vi "MoveCarriageToPosition.vi"(6 "Lift Speed":dbl, 7 "Target Height":dbl) -> ()   [LabVIEW 2017]
uses:
  Robot Global Data.vi
  <vilib>/Rock Robotics/Network Tables/NT Write Number.vi
  <vilib>/addons/control/pid/pid.llb/PID (DBL).vi
  <vilib>/addons/control/pid/NI_PID_pid.lvlib
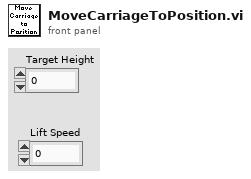
[diagram p1: front panel]
types:
  T1 = cluster{"proportional gain (Kc)":dbl, "integral time (Ti, min)":dbl, "derivative time (Td, min)":dbl}
  T2 = typedef "WPI_MotorControlDeviceRef.ctl" = cluster{"DeviceStatus":errorcluster, "Type":T3, "PWM":cluster{"PWM Channel":T4, "DeadBand":T5}, "CAN":cluster{"Device Number":u8, "SetOutput VI Ref":variant, "GetOutput VI Ref":variant, "Enable VI Ref":variant, "Disable VI Ref":variant, "Data":variant}, "Invert":bool, "DIO PWM":cluster{"PWM \"Enable\" Channel":T4, "DIOChannel":T6, "PWM Rate":dbl}}
  T3 = typedef "WPI_MotorControlType.ctl" = enum16{"PWM", "CAN", "DIO PWM"}
  T4 = typedef "FPGA_DIOPWMChannel.ctl" = enum8{"PWM 0", "PWM 1", "PWM 2", "PWM 3", "PWM 4", "PWM 5", "PWM 6", "PWM 7", "PWM 8", "PWM 9", "PWM MXP 0", "PWM MXP 1", "PWM MXP 2", "PWM MXP 3", "PWM MXP 4", "PWM MXP 5", "PWM MXP 6", "PWM MXP 7", "PWM MXP 8", "PWM MXP 9", "Invalid"}
  T5 = typedef "WPI_PWMDeadband.ctl" = cluster{"Name":string, "maxPositivePwm":i32, "minPositivePwm":i32, "centerPwm":i32, "maxNegativePwm":i32, "minNegativePwm":i32, "angularRange":u16}
  T6 = typedef "FPGA_DIOChannel.ctl" = enum8{"DIO 0", "DIO 1", "DIO 2", "DIO 3", "DIO 4", "DIO 5", "DIO 6", "DIO 7", "DIO 8", "DIO 9", "DIO MXP 0", "DIO MXP 1", "DIO MXP 2", "DIO MXP 3", "DIO MXP 4", "DIO MXP 5", "DIO MXP 6", "DIO MXP 7", "DIO MXP 8", "DIO MXP 9", "DIO MXP 10", "DIO MXP 11", "DIO MXP 12", "DIO MXP 13", "DIO MXP 14", "DIO MXP 15", "SPI Port CS1", "SPI Port CS2", "SPI Port CS3", "SPI Port MISO", "SPI Port MOSI", "Invalid"}
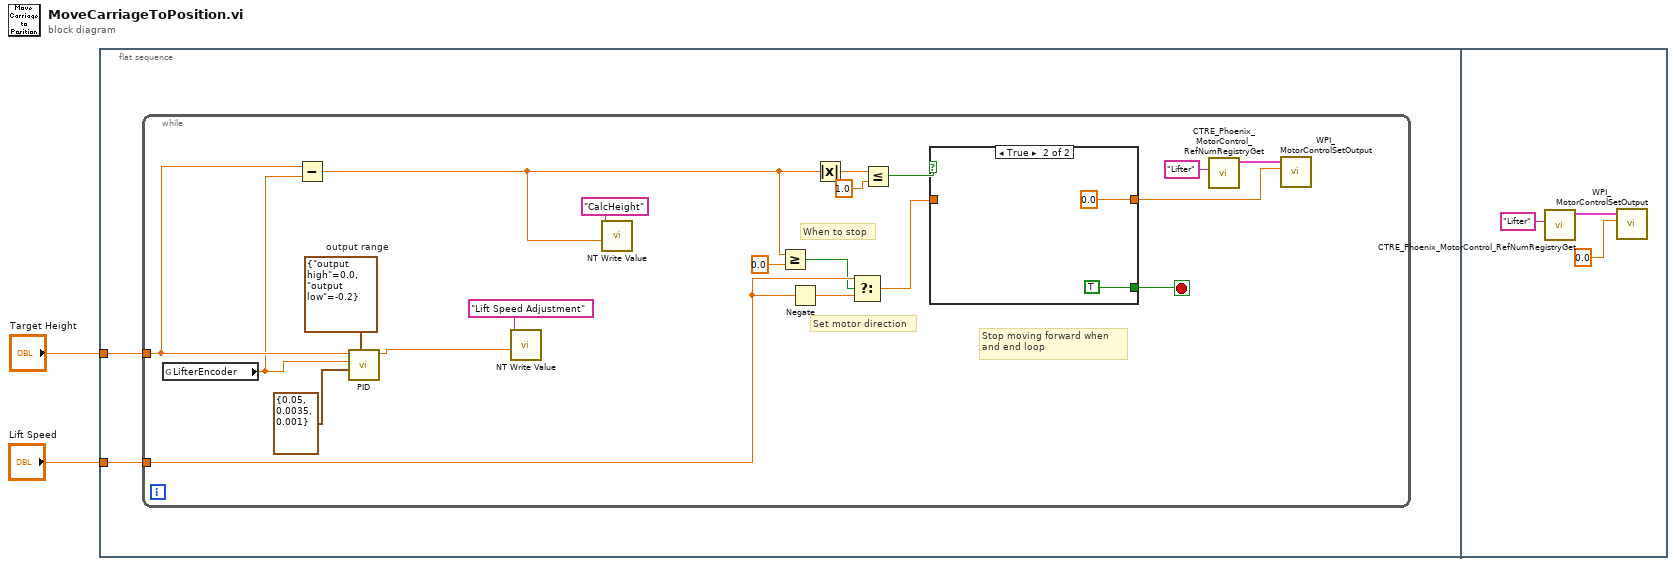
[diagram p0: block diagram]
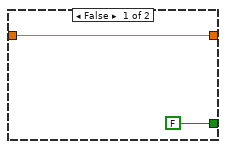
[diagram p2: hidden frame]
diagram:
  n1 = flat-sequence {
    tunnel: "Target Height" -> [w3]
    tunnel: "Lift Speed" -> [w4]
    frame #0 {
      n2 = while {
        tunnel: w4 -> [w13]
        tunnel: w3 -> [w21]
        stop <- w24 stop-if-true
        w22 = cluster{"output high":dbl, "output low":dbl} {"output high"=0.0, "output low"=-0.2}  # output range
        # "Set motor direction"
        # "When to stop"
        # "Stop moving forward when\nand end loop"
        n3 = global read "Robot Global Data.vi" "LifterEncoder"() -> (w20:dbl)
        n4 = Subtract(x=w21, y=w20) -> (x-y=w5:dbl)
        n5 = call-poly <vilib>:"PID.vi"("output range"=w22, "PID gains"=T1 {"proportional gain (Kc)"=0.05, "integral time (Ti, min)"=0.0035, "derivative time (Td, min)"=0.001}, "process variable"=w20, "setpoint"=w21) -> ("output"=w10:dbl)  [unwired: 6 in, 1 out]
        n6 = call-poly <vilib>:"NT Write Value.vi"("Numeric"=w10, "Name"="Lift Speed Adjustment") -> ()  [unwired: 9 in, 1 out]
        n7 = call-poly <vilib>:"NT Write Value.vi"("Numeric"=w5, "Name"="CalcHeight") -> ()  [unwired: 9 in, 1 out]
        n8 = Greater Or Equal?(x=w5, y=0.0) -> (x >= y?=w11:bool)
        n9 = Negate(x=w13) -> (-x=w14:dbl)
        n10 = Absolute Value(x=w5) -> (abs(x)=w8:dbl)
        n11 = Select(t=w13, s=w11, f=w14) -> (s? t:f=w15:dbl)
        n12 = Less Or Equal?(x=w8, y=1.0) -> (x <= y?=w19:bool)
        n13 = case shown="True" w19 {
          tunnel: [FALSE TRUE] -> w24
          tunnel: w15 -> [w25 _]
          tunnel: [w25 0.0] -> w16
          frame False {
          }
          frame True {
          }
        }
        n14 = call <vilib>:"CTRE_Phoenix_MotorControl_RefNumRegistryGet.vi"("refnum name"="Lifter") -> ("PhoenixMotorControlDevRef"=w17:T2)  [unwired: 9 in, 1 out]
        n15 = call <vilib>:"WPI_MotorControlSetOutput.vi"("Output"=w16, "MotorControlDevRef"=w17) -> ()  [unwired: 7 in, 3 out]
      }
    }
    frame #1 {
      n16 = call <vilib>:"CTRE_Phoenix_MotorControl_RefNumRegistryGet.vi"("refnum name"="Lifter") -> ("PhoenixMotorControlDevRef"=w30:T2)  [unwired: 9 in, 1 out]
      n17 = call <vilib>:"WPI_MotorControlSetOutput.vi"("Output"=0.0, "MotorControlDevRef"=w30) -> ()  [unwired: 7 in, 3 out]
    }
  }
